vi "merFISH_create_tasks_list_TDMS.vi"(2 "Injection procedure empty?":bool, 3 "merFISH mode":u16, 4 "error in":errorcluster, 5 "merFISH path":path=path "E:/", 6 "Probe List Refnum":refnum<vi>, 7 "XY positions":dbl[][](array[numeric])) -> (0 "error out":errorcluster, 1 "refnum log file":refnum<file>)   [LabVIEW 2015]
uses:
  CONTROLS/Q_main_element.ctl
  GLOBAL/Global_MAIN.vi
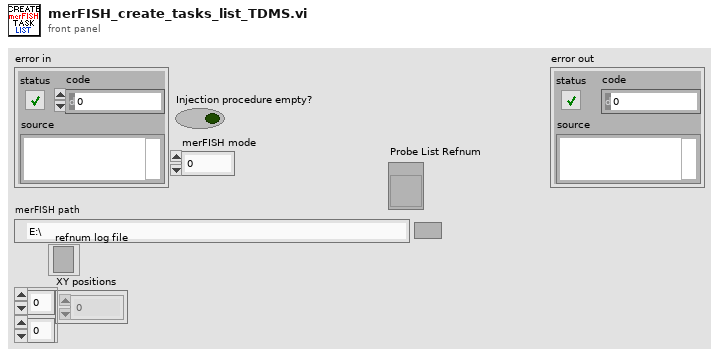
[diagram p1: front panel]
types:
  T1 = typedef "Q_main_element.ctl" = cluster{"variant":variant, "Instruction":enum16{"Main_idle", "Main_initialize", "Main_initialize_TDMS", "Main_initialize_Queue", "Main_error", "Main_DAQ_initialization_results", "Main_ASI_initialization_results", "Main_Piezo_initialization_results", "Main_Valve_initialization_results", "Main_Pump_initialization_results", "Main_CAMERA_initialization_results", "Main_FPGA_initialization_results", "Main_DAQ_error", "Main_ASI_error", "Main_Piezo_error", "Main_CAMERA_error", "Main_Valve_error", "Main_Pump_error", "Main_FPGA_error", "Main_start_acquiring", "Main_not_acquiring", "Main_acquiring", "Main_stop_acquiring", "Main_change_exposure", "Main_change_z_scan_parameters", "Main_define_ROI", "Main_define_mosaic", "Main_read_kinetic_time", "Main_cooler", "Main_read_temperature", "Main_save_XY", "Main_load_XY", "Main_discard_XY", "Main_move_to_XY", "Main_measure_QPD", "Main_autofocus_calibration", "Main_autofocus_initialization", "Main_autofocus_stop", "Main_save_PID", "Main_change_H_valve_position", "Main_two_way_valve", "Main_save_movie", "Main_init_single_scan", "Main_single_scan", "Main_stop_single_scan", "Main_merFISH_illumination_parameters", "Main_merFISH_buffer_probe_list", "Main_merFISH_injections_procedure", "Main_merFISH_save_setpoint", "Main_merFISH_DAPI_parameters", "Main_merFISH_Brightfield_parameters", "Main_merFISH_save_embryo_ROI", "Main_merFISH_init", "Main_merFISH_resume", "Main_merFISH_start_autofocus", "Main_merFISH_open_close_valve_merFISH", "Main_merFISH_open_close_valve_photobleaching", "Main_merFISH_hybridization", "Main_merFISH_move_to_ROI", "Main_merFISH_wait_stabilization", "Main_merFISH_move_to_REF", "Main_merFISH_scan", "Main_merFISH_photobleaching_injection", "Main_merFISH_photobleaching", "Main_merFISH_send_email", "Main_merFISH_close", "Main_STOP"}}
  T2 = enum16{"open", "replace", "create", "open or create", "replace or create", "replace or create with confirmation"}
  T3 = enum16{"Single ROIs & no injection", "Single ROIs & injections", "Embryos & no injection", "Embryos & injections"}
  T4 = cluster{"ROI #":i32, "Probe #":i32, "Folder# ":i32, "Embryo #":i32}
  T5 = enum16{"open", "open or create", "create or replace", "create", "open (read-only)"}
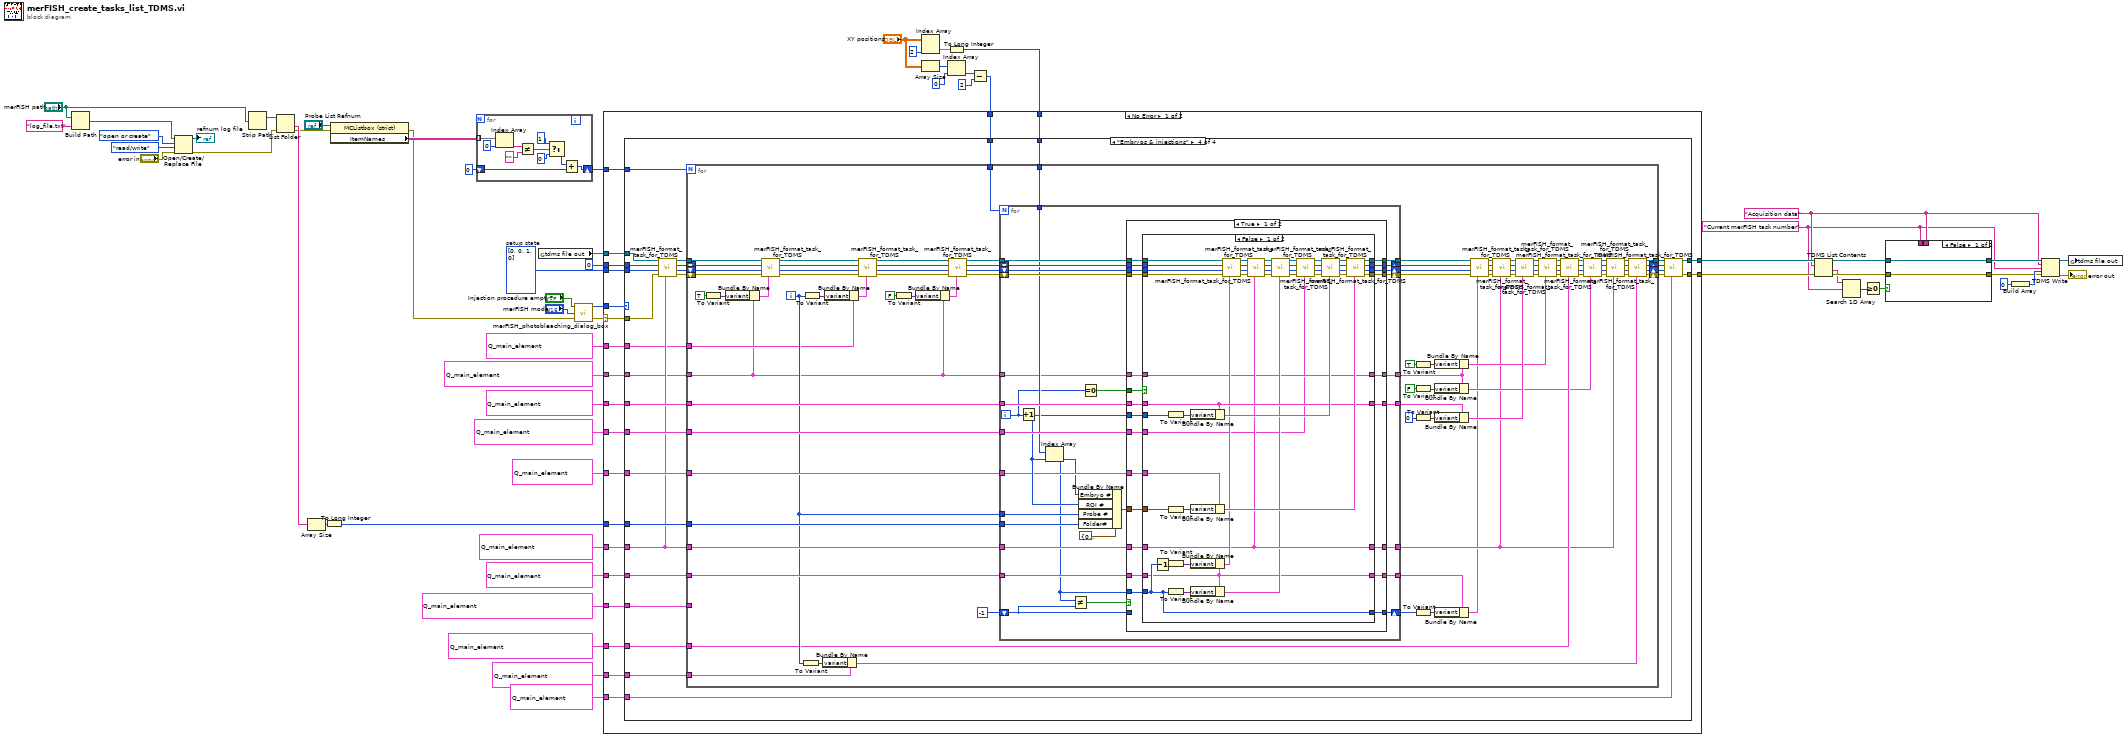
[diagram p0: block diagram]
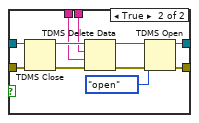
[diagram p2: hidden frame]
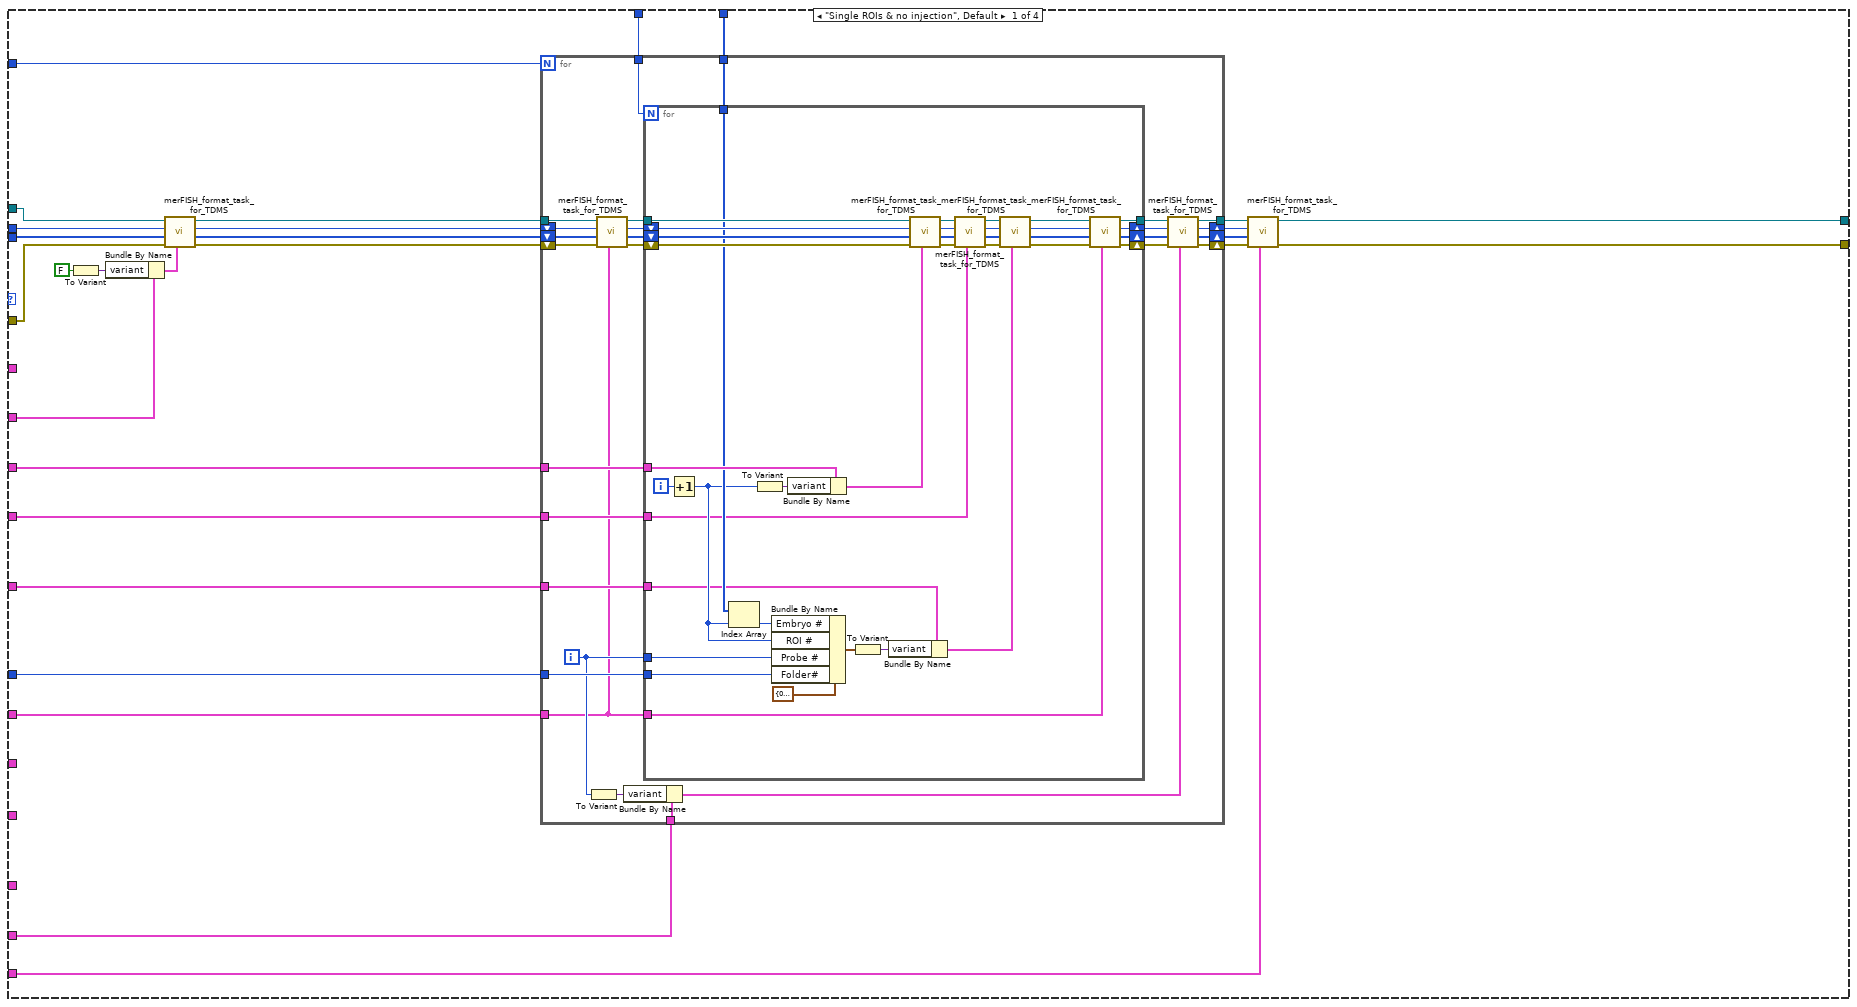
[diagram p3: hidden frame]
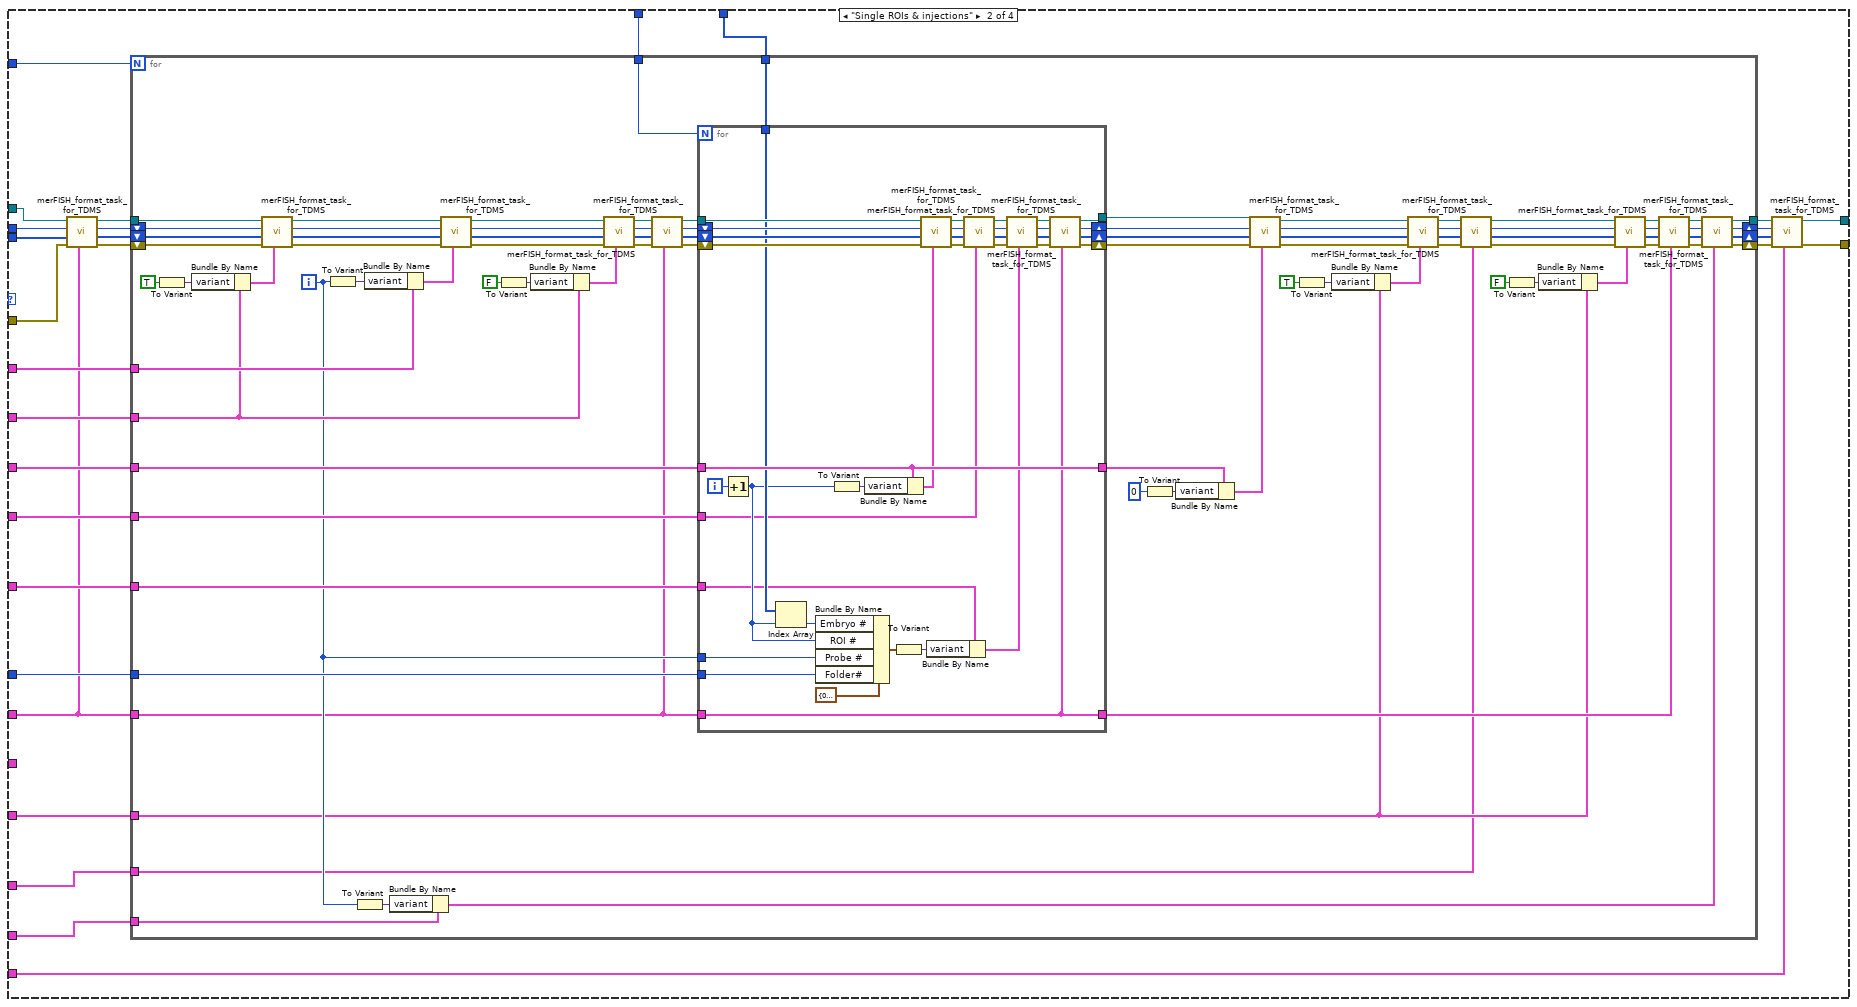
[diagram p4: hidden frame]
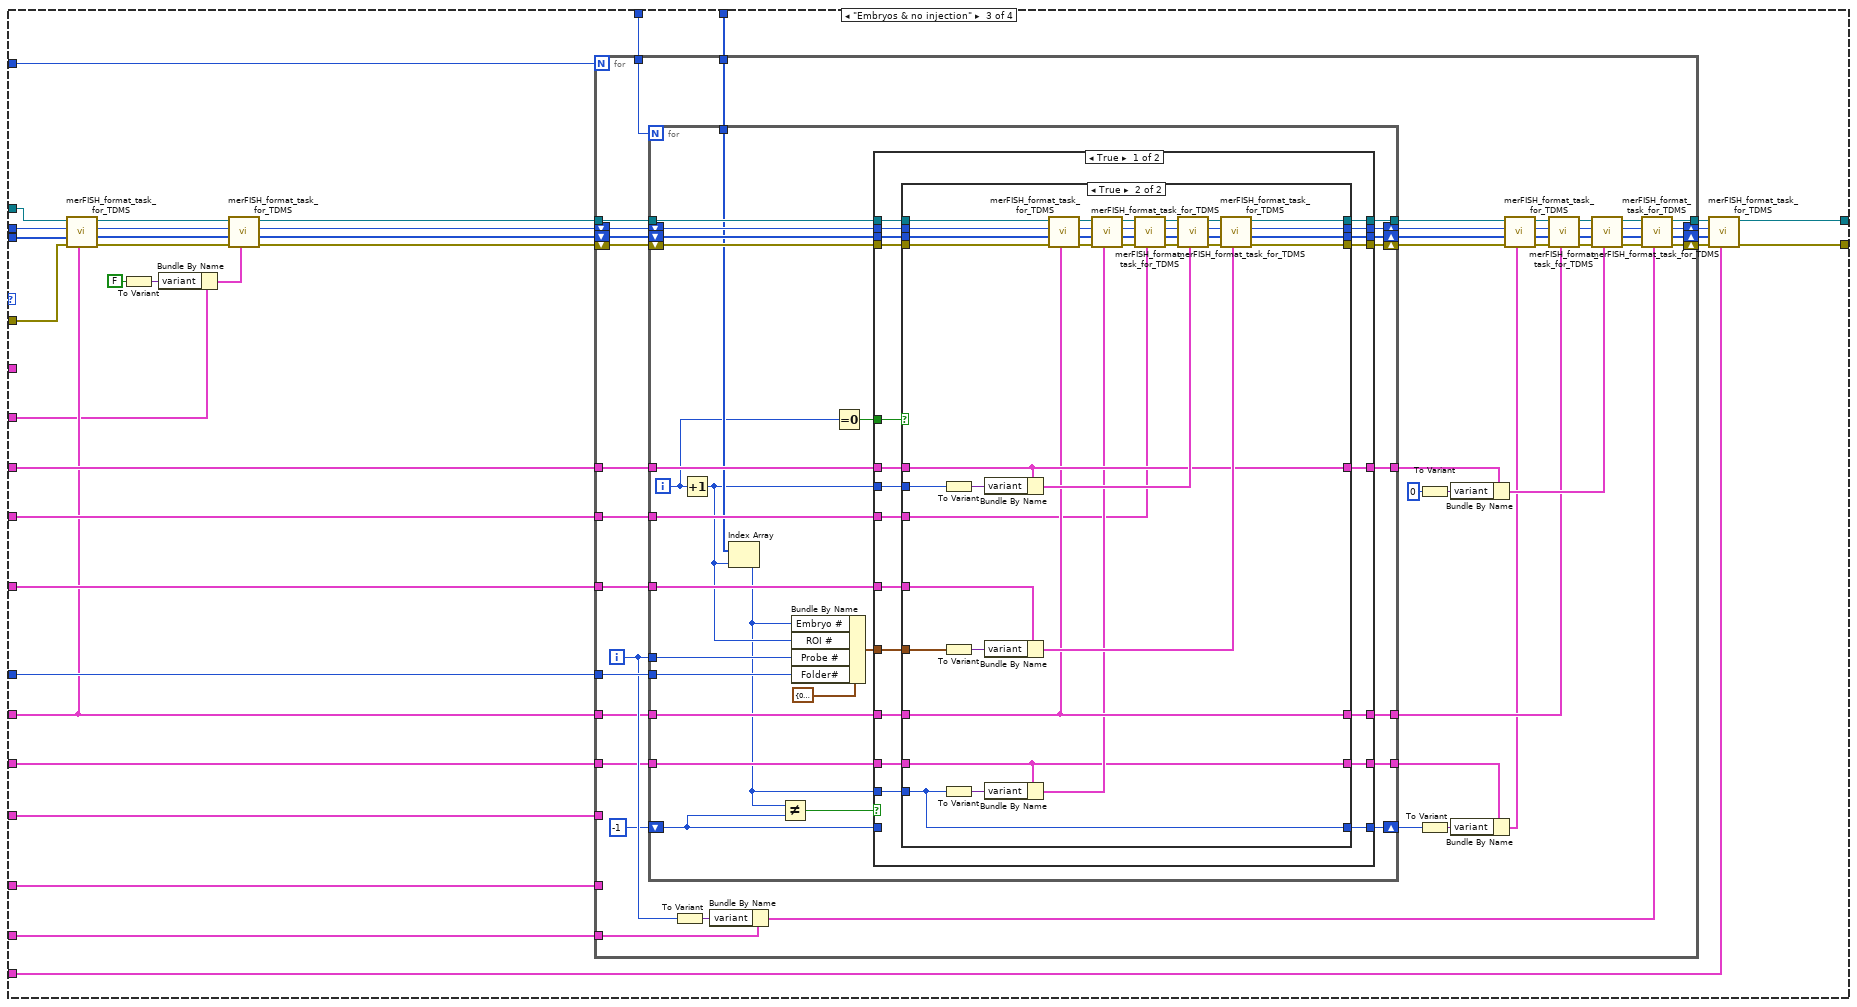
[diagram p5: hidden frame]
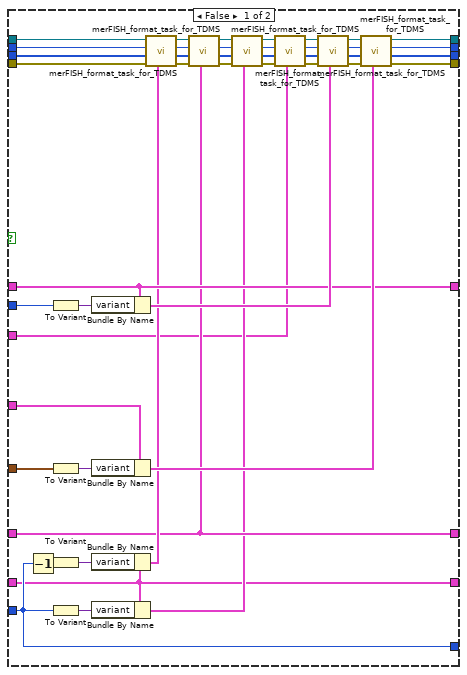
[diagram p6: hidden frame]
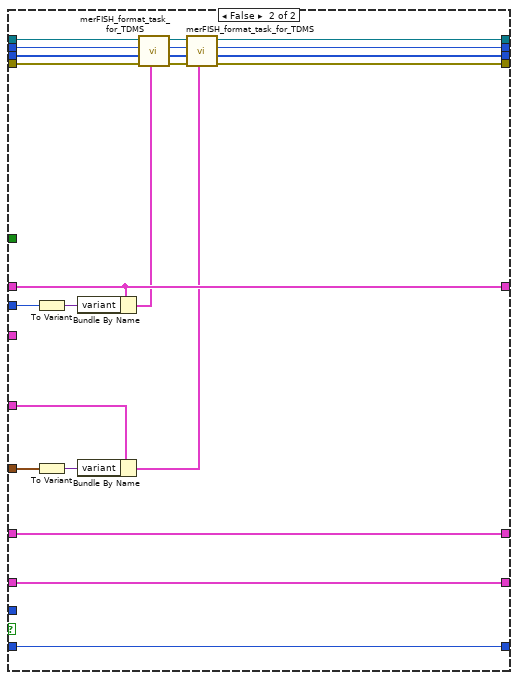
[diagram p7: hidden frame]
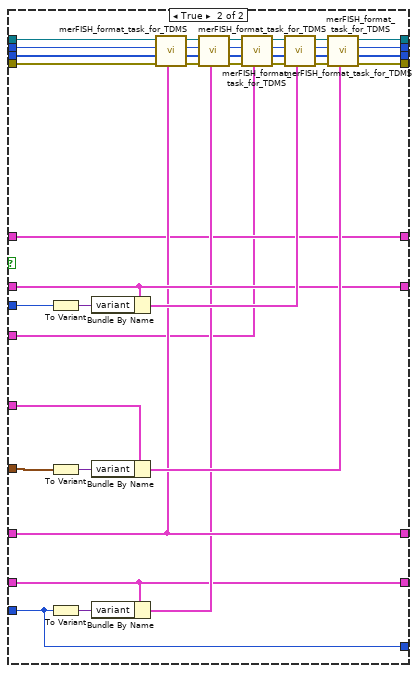
[diagram p8: hidden frame]
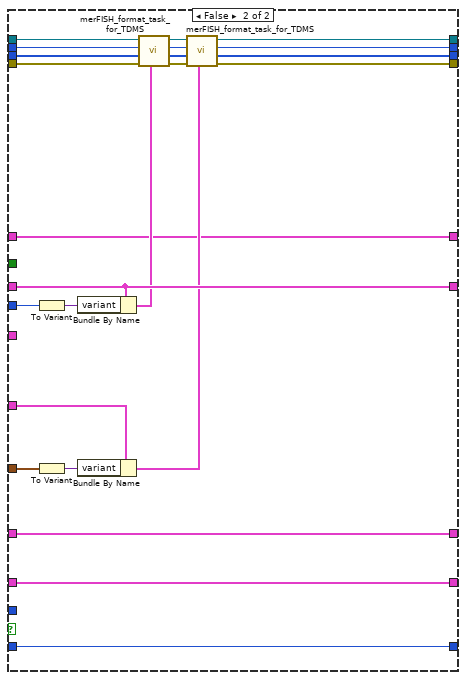
[diagram p9: hidden frame]
diagram:
  w13 = i32[] [0, 0, 1, 0]  # setup state
  w18 = "Current merFISH task number" ("group name in")
  w19 = "Acquisition data" ("group name in")
  n1 = Build Path(base path="merFISH path", name or relative path="log_file.txt") -> (appended path=w42:path)
  n2 = Open/Create/Replace File(file path (use dialog)=w42, error in="error in", operation (0:open)=T2."open or create", access (0:read/write)=enum16{"read/write", "read-only", "write-only"}."read/write") -> (refnum out=→"refnum log file":refnum<file>, error out=w37:errorcluster)  [unwired: 2 in, 1 out]
  n3 = Strip Path(path="merFISH path") -> (stripped path=w36:path)  [unwired: 1 out]
  n4 = List Folder(path=w36, error in=w37) -> (folder names=w50:string[], error out=w48:errorcluster)  [unwired: 2 in, 2 out]
  n5 = Array Size(array=w50) -> (size(s)=w49:i32)
  n6 = To Long Integer(number=w49) -> (32bit integer=w47:i32)
  n7 = property class="MCListbox (strict)"(reference="Probe List Refnum", error in=w48) -> (error out=w31:errorcluster, "ItemNames"=w53:string[][])  [unwired: 1 out]
  n8 = for {
    tunnel: w53 -> [w70] mode=indexing
    shift-right: [w63] -> w51
    shift-left: 0 ("f") -> [w61]
    n9 = Index Array(array=w70, index=0) -> (element=w68:string)
    n10 = Not Equal?(x=w68, y="") -> (x != y?=w66:bool)
    n11 = Select(t=1, s=w66, f=0) -> (s? t:f=w62:i32)
    n12 = Add(x=w62, y=w61) -> (x+y=w63:i32)
  }
  n13 = global read "Global_MAIN.vi" "tdms file out"() -> (w29:refnum<k34>)
  n14 = call "merFISH_photobleaching_dialog_box.vi"("error in"=w31, "merFISH mode"="merFISH mode", "Injection procedure empty?"="Injection procedure empty?") -> ("error out"=w35:errorcluster, "Which experiment?"=w34:T3)  [unwired: 1 in]
  n15 = Index Array(array="XY positions", index (col)=2 ("disabled index (col)")) -> (element=w4:dbl[])  [unwired: 1 in]
  n16 = Array Size(array="XY positions") -> (size(s)=w10:i32[])
  n17 = To Long Integer(number=w4) -> (32bit integer=w3:i32[])
  n18 = Index Array(array=w10, index=0) -> (element=w9:i32)
  n19 = Subtract(x=w9, y=2) -> (x-y=w7:i32)
  n20 = case shown="No Error" w35 {
    selector: w35 -> [w79 w850]
    tunnel: T1 {"variant"=variant, "Instruction"=enum."Main_merFISH_move_to_ROI"} ("element") -> [w92 _]
    tunnel: T1 {"variant"=variant, "Instruction"=enum."Main_merFISH_wait_stabilization"} ("element") -> [w91 _]
    tunnel: T1 {"variant"=variant, "Instruction"=enum."Main_merFISH_scan"} ("element") -> [w90 _]
    tunnel: T1 {"variant"=variant, "Instruction"=enum."Main_merFISH_close"} ("element") -> [w89 _]
    tunnel: T1 {"variant"=variant, "Instruction"=enum."Main_merFISH_start_autofocus"} ("element") -> [w88 _]
    tunnel: T1 {"variant"=variant, "Instruction"=enum."Main_merFISH_hybridization"} ("element") -> [w87 _]
    tunnel: w51 -> [w86 _]
    tunnel: w47 -> [w85 _]
    tunnel: T1 {"variant"=variant, "Instruction"=enum."Main_merFISH_open_close_valve_merFISH"} ("element") -> [w84 _]
    tunnel: w34 -> [w83 _]
    tunnel: T1 {"variant"=variant, "Instruction"=enum."Main_merFISH_photobleaching_injection"} ("element") -> [w82 _]
    tunnel: T1 {"variant"=variant, "Instruction"=enum."Main_merFISH_send_email"} ("element") -> [w81 _]
    tunnel: T1 {"variant"=variant, "Instruction"=enum."Main_merFISH_open_close_valve_photobleaching"} ("element") -> [w80 _]
    tunnel: 0 ("index") -> [w78 _]
    tunnel: [w77 w850] -> w21
    tunnel: w29 -> [w76 w849]
    tunnel: [w75 w849] -> w20
    tunnel: w13 -> [w74 _]
    tunnel: w7 -> [w73 _]
    tunnel: w3 -> [w72 _]
    tunnel: T1 {"variant"=variant, "Instruction"=enum."Main_merFISH_move_to_REF"} ("element") -> [w71 _]
    frame No Error {
      n21 = case shown="\"Embryos & injections\"" w83 {
        tunnel: w92 -> [w120 w208 w363 w593]
        tunnel: w91 -> [w119 w207 w362 w592]
        tunnel: w90 -> [w118 w206 w361 w591]
        tunnel: w89 -> [w111 w196 w353 w583]
        tunnel: w88 -> [w114 w201 w356 w586]
        tunnel: w87 -> [_ w210 _ w566]
        tunnel: w86 -> [w117 w211 w364 w594]
        tunnel: w85 -> [w116 w205 w360 w590]
        tunnel: w84 -> [w93 w209 w335 w567]
        tunnel: w82 -> [_ w203 w358 w588]
        tunnel: w81 -> [w115 w204 w359 w589]
        tunnel: w80 -> [_ w184 w343 w573]
        tunnel: w79 -> [w94 w202 w357 w587]
        tunnel: [w110 w195 w352 w582] -> w77
        tunnel: w78 -> [w99 w194 w351 w581]
        tunnel: w76 -> [w101 w193 w350 w580]
        tunnel: [w108 w190 w348 w578] -> w75
        tunnel: w74 -> [w95 w189 w347 w577]
        tunnel: w73 -> [w106 w186 w345 w575]
        tunnel: w72 -> [w105 w185 w344 w574]
        tunnel: w71 -> [_ _ w330 w572]
        frame "Single ROIs & no injection", Default {
          n22 = To Variant(anything=FALSE) -> (Variant=w104:variant)
          n23 = Bundle By Name(cluster=w93, "variant"=w104) -> (w102:T1)
          n24 = call "merFISH_format_task_for_TDMS.vi"("Task"=w102, "error in"=w94, "setup state"=w95, "Task number"=w99, "tdms file"=w101) -> ("error out"=w96:errorcluster, "setup state out"=w97:i32[], "Next task number"=w98:i32, "tdms file out"=w100:refnum<k34>)
          n25 = for {
            N: w117 -> [_]
            tunnel: w120 -> [w147]
            tunnel: w119 -> [w146]
            tunnel: w118 -> [w145]
            tunnel: w114 -> [w140]
            tunnel: w116 -> [w144]
            tunnel: w115 -> [w141]
            shift-right: [w134] -> w113
            shift-left: w98 -> [w124]
            shift-right: [w133] -> w112
            shift-left: w96 -> [w121]
            tunnel: w100 -> [w123]
            tunnel: [w130] -> w109
            shift-right: [w127] -> w107
            shift-left: w97 -> [w122]
            tunnel: w106 -> [w126]
            tunnel: w105 -> [w125]
            i -> [w142]
            n26 = To Variant(anything=w142) -> (Variant=w143:variant)
            n27 = call "merFISH_format_task_for_TDMS.vi"("Task"=w140, "error in"=w121, "setup state"=w122, "Task number"=w124, "tdms file"=w123) -> ("error out"=w138:errorcluster, "setup state out"=w129:i32[], "Next task number"=w139:i32, "tdms file out"=w132:refnum<k34>)
            n28 = Bundle By Name(cluster=w141, "variant"=w143) -> (w135:T1)
            n29 = for {
              N: w126 -> [_]
              tunnel: w147 -> [w182]
              tunnel: w146 -> [w148]
              tunnel: w145 -> [w157]
              tunnel: w140 -> [w171]
              tunnel: w142 -> [w180]
              tunnel: w144 -> [w179]
              shift-right: [w151] -> w137
              shift-left: w139 -> [w178]
              shift-right: [w149] -> w136
              shift-left: w138 -> [w177]
              tunnel: w132 -> [w170]
              tunnel: [w152] -> w131
              shift-right: [w150] -> w128
              shift-left: w129 -> [w167]
              tunnel: w125 -> [w163]
              i -> [w181]
              n30 = Increment(x=w181) -> (x+1=w162:i32)
              n31 = Index Array(array=w163, index=w162) -> (element=w161:i32)
              n32 = To Variant(anything=w162) -> (Variant=w183:variant)
              n33 = Bundle By Name(cluster=T4 {"ROI #"=0, "Probe #"=0, "Folder# "=0, "Embryo #"=0}, "Embryo #"=w161, "ROI #"=w162, "Probe #"=w180, "Folder#"=w179) -> (w160:T4)
              n34 = Bundle By Name(cluster=w182, "variant"=w183) -> (w176:T1)
              n35 = To Variant(anything=w160) -> (Variant=w158:variant)
              n36 = Bundle By Name(cluster=w157, "variant"=w158) -> (w159:T1)
              n37 = call "merFISH_format_task_for_TDMS.vi"("Task"=w176, "error in"=w177, "setup state"=w167, "Task number"=w178, "tdms file"=w170) -> ("error out"=w174:errorcluster, "setup state out"=w166:i32[], "Next task number"=w175:i32, "tdms file out"=w169:refnum<k34>)
              n38 = call "merFISH_format_task_for_TDMS.vi"("Task"=w148, "error in"=w174, "setup state"=w166, "Task number"=w175, "tdms file"=w169) -> ("error out"=w172:errorcluster, "setup state out"=w165:i32[], "Next task number"=w173:i32, "tdms file out"=w168:refnum<k34>)
              n39 = call "merFISH_format_task_for_TDMS.vi"("Task"=w159, "error in"=w172, "setup state"=w165, "Task number"=w173, "tdms file"=w168) -> ("error out"=w153:errorcluster, "setup state out"=w154:i32[], "Next task number"=w155:i32, "tdms file out"=w156:refnum<k34>)
              n40 = call "merFISH_format_task_for_TDMS.vi"("Task"=w171, "error in"=w153, "setup state"=w154, "Task number"=w155, "tdms file"=w156) -> ("error out"=w149:errorcluster, "setup state out"=w150:i32[], "Next task number"=w151:i32, "tdms file out"=w152:refnum<k34>)
            }
            n41 = call "merFISH_format_task_for_TDMS.vi"("Task"=w135, "error in"=w136, "setup state"=w128, "Task number"=w137, "tdms file"=w131) -> ("error out"=w133:errorcluster, "setup state out"=w127:i32[], "Next task number"=w134:i32, "tdms file out"=w130:refnum<k34>)
          }
          n42 = call "merFISH_format_task_for_TDMS.vi"("Task"=w111, "error in"=w112, "setup state"=w107, "Task number"=w113, "tdms file"=w109) -> ("error out"=w110:errorcluster, "tdms file out"=w108:refnum<k34>)  [unwired: 2 out]
        }
        frame "Single ROIs & injections" {
          n43 = call "merFISH_format_task_for_TDMS.vi"("Task"=w201, "error in"=w202, "setup state"=w189, "Task number"=w194, "tdms file"=w193) -> ("error out"=w199:errorcluster, "setup state out"=w188:i32[], "Next task number"=w200:i32, "tdms file out"=w192:refnum<k34>)
          n44 = for {
            N: w211 -> [_]
            tunnel: w208 -> [w293]
            tunnel: w207 -> [w292]
            tunnel: w206 -> [w291]
            tunnel: w201 -> [w261]
            tunnel: w210 -> [w284]
            tunnel: w205 -> [w289]
            tunnel: w209 -> [w279]
            tunnel: w184 -> [w213]
            tunnel: w204 -> [w274]
            tunnel: w203 -> [w212]
            shift-right: [w243] -> w197
            shift-left: w199 -> [w271]
            shift-right: [w242] -> w198
            shift-left: w200 -> [w272]
            tunnel: w192 -> [w241]
            tunnel: [w230] -> w191
            shift-right: [w218] -> w187
            shift-left: w188 -> [w229]
            tunnel: w186 -> [w217]
            tunnel: w185 -> [w216]
            i -> [w273]
            n45 = To Variant(anything=TRUE) -> (Variant=w288:variant)
            n46 = Bundle By Name(cluster=w279, "variant"=w288) -> (w270:T1)
            n47 = call "merFISH_format_task_for_TDMS.vi"("Task"=w270, "error in"=w271, "setup state"=w229, "Task number"=w272, "tdms file"=w241) -> ("error out"=w268:errorcluster, "setup state out"=w228:i32[], "Next task number"=w269:i32, "tdms file out"=w240:refnum<k34>)
            n48 = To Variant(anything=w273) -> (Variant=w290:variant)
            n49 = To Variant(anything=w273) -> (Variant=w275:variant)
            n50 = Bundle By Name(cluster=w284, "variant"=w290) -> (w267:T1)
            n51 = Bundle By Name(cluster=w274, "variant"=w275) -> (w215:T1)
            n52 = call "merFISH_format_task_for_TDMS.vi"("Task"=w267, "error in"=w268, "setup state"=w228, "Task number"=w269, "tdms file"=w240) -> ("error out"=w265:errorcluster, "setup state out"=w227:i32[], "Next task number"=w266:i32, "tdms file out"=w239:refnum<k34>)
            n53 = To Variant(anything=FALSE) -> (Variant=w285:variant)
            n54 = Bundle By Name(cluster=w279, "variant"=w285) -> (w264:T1)
            n55 = call "merFISH_format_task_for_TDMS.vi"("Task"=w264, "error in"=w265, "setup state"=w227, "Task number"=w266, "tdms file"=w239) -> ("error out"=w262:errorcluster, "setup state out"=w226:i32[], "Next task number"=w263:i32, "tdms file out"=w238:refnum<k34>)
            n56 = call "merFISH_format_task_for_TDMS.vi"("Task"=w261, "error in"=w262, "setup state"=w226, "Task number"=w263, "tdms file"=w238) -> ("error out"=w260:errorcluster, "setup state out"=w225:i32[], "Next task number"=w259:i32, "tdms file out"=w237:refnum<k34>)
            n57 = for {
              N: w217 -> [_]
              tunnel: w293 -> [w325]
              tunnel: w292 -> [w294]
              tunnel: w291 -> [w301]
              tunnel: w261 -> [w317]
              tunnel: w273 -> [w327]
              tunnel: w289 -> [w326]
              tunnel: [w325] -> w277
              tunnel: [w317] -> w248
              shift-right: [w315] -> w258
              shift-left: w259 -> [w324]
              shift-right: [w316] -> w257
              shift-left: w260 -> [w323]
              tunnel: w237 -> [w314]
              tunnel: [w311] -> w236
              shift-right: [w307] -> w224
              shift-left: w225 -> [w310]
              tunnel: w216 -> [w304]
              i -> [w328]
              n58 = Increment(x=w328) -> (x+1=w303:i32)
              n59 = Index Array(array=w304, index=w303) -> (element=w305:i32)
              n60 = Bundle By Name(cluster=T4 {"ROI #"=0, "Probe #"=0, "Folder# "=0, "Embryo #"=0}, "Embryo #"=w305, "ROI #"=w303, "Probe #"=w327, "Folder#"=w326) -> (w300:T4)
              n61 = To Variant(anything=w303) -> (Variant=w329:variant)
              n62 = Bundle By Name(cluster=w325, "variant"=w329) -> (w322:T1)
              n63 = To Variant(anything=w300) -> (Variant=w302:variant)
              n64 = call "merFISH_format_task_for_TDMS.vi"("Task"=w322, "error in"=w323, "setup state"=w310, "Task number"=w324, "tdms file"=w314) -> ("error out"=w320:errorcluster, "setup state out"=w309:i32[], "Next task number"=w321:i32, "tdms file out"=w313:refnum<k34>)
              n65 = Bundle By Name(cluster=w301, "variant"=w302) -> (w299:T1)
              n66 = call "merFISH_format_task_for_TDMS.vi"("Task"=w294, "error in"=w320, "setup state"=w309, "Task number"=w321, "tdms file"=w313) -> ("error out"=w319:errorcluster, "setup state out"=w308:i32[], "Next task number"=w318:i32, "tdms file out"=w312:refnum<k34>)
              n67 = call "merFISH_format_task_for_TDMS.vi"("Task"=w299, "error in"=w319, "setup state"=w308, "Task number"=w318, "tdms file"=w312) -> ("error out"=w295:errorcluster, "setup state out"=w296:i32[], "Next task number"=w297:i32, "tdms file out"=w298:refnum<k34>)
              n68 = call "merFISH_format_task_for_TDMS.vi"("Task"=w317, "error in"=w295, "setup state"=w296, "Task number"=w297, "tdms file"=w298) -> ("error out"=w316:errorcluster, "setup state out"=w307:i32[], "Next task number"=w315:i32, "tdms file out"=w311:refnum<k34>)
            }
            n69 = To Variant(anything=0) -> (Variant=w278:variant)
            n70 = Bundle By Name(cluster=w277, "variant"=w278) -> (w256:T1)
            n71 = call "merFISH_format_task_for_TDMS.vi"("Task"=w256, "error in"=w257, "setup state"=w224, "Task number"=w258, "tdms file"=w236) -> ("error out"=w254:errorcluster, "setup state out"=w223:i32[], "Next task number"=w255:i32, "tdms file out"=w235:refnum<k34>)
            n72 = To Variant(anything=TRUE) -> (Variant=w283:variant)
            n73 = Bundle By Name(cluster=w213, "variant"=w283) -> (w214:T1)
            n74 = call "merFISH_format_task_for_TDMS.vi"("Task"=w214, "error in"=w254, "setup state"=w223, "Task number"=w255, "tdms file"=w235) -> ("error out"=w253:errorcluster, "setup state out"=w222:i32[], "Next task number"=w252:i32, "tdms file out"=w234:refnum<k34>)
            n75 = call "merFISH_format_task_for_TDMS.vi"("Task"=w212, "error in"=w253, "setup state"=w222, "Task number"=w252, "tdms file"=w234) -> ("error out"=w250:errorcluster, "setup state out"=w221:i32[], "Next task number"=w251:i32, "tdms file out"=w233:refnum<k34>)
            n76 = To Variant(anything=FALSE) -> (Variant=w280:variant)
            n77 = Bundle By Name(cluster=w213, "variant"=w280) -> (w249:T1)
            n78 = call "merFISH_format_task_for_TDMS.vi"("Task"=w249, "error in"=w250, "setup state"=w221, "Task number"=w251, "tdms file"=w233) -> ("error out"=w247:errorcluster, "setup state out"=w220:i32[], "Next task number"=w246:i32, "tdms file out"=w232:refnum<k34>)
            n79 = call "merFISH_format_task_for_TDMS.vi"("Task"=w248, "error in"=w247, "setup state"=w220, "Task number"=w246, "tdms file"=w232) -> ("error out"=w244:errorcluster, "setup state out"=w219:i32[], "Next task number"=w245:i32, "tdms file out"=w231:refnum<k34>)
            n80 = call "merFISH_format_task_for_TDMS.vi"("Task"=w215, "error in"=w244, "setup state"=w219, "Task number"=w245, "tdms file"=w231) -> ("error out"=w243:errorcluster, "setup state out"=w218:i32[], "Next task number"=w242:i32, "tdms file out"=w230:refnum<k34>)
          }
          n81 = call "merFISH_format_task_for_TDMS.vi"("Task"=w196, "error in"=w197, "setup state"=w187, "Task number"=w198, "tdms file"=w191) -> ("error out"=w195:errorcluster, "tdms file out"=w190:refnum<k34>)  [unwired: 2 out]
        }
        frame "Embryos & no injection" {
          n82 = call "merFISH_format_task_for_TDMS.vi"("Task"=w356, "error in"=w357, "setup state"=w347, "Task number"=w351, "tdms file"=w350) -> ("error out"=w336:errorcluster, "setup state out"=w337:i32[], "Next task number"=w338:i32, "tdms file out"=w339:refnum<k34>)
          n83 = To Variant(anything=FALSE) -> (Variant=w342:variant)
          n84 = Bundle By Name(cluster=w335, "variant"=w342) -> (w340:T1)
          n85 = call "merFISH_format_task_for_TDMS.vi"("Task"=w340, "error in"=w336, "setup state"=w337, "Task number"=w338, "tdms file"=w339) -> ("error out"=w331:errorcluster, "setup state out"=w332:i32[], "Next task number"=w333:i32, "tdms file out"=w334:refnum<k34>)
          n86 = for {
            N: w364 -> [_]
            tunnel: w363 -> [w410]
            tunnel: w362 -> [w409]
            tunnel: w361 -> [w408]
            tunnel: w356 -> [w400]
            tunnel: w360 -> [w407]
            tunnel: w343 -> [_]
            tunnel: w359 -> [w402]
            tunnel: w358 -> [_]
            shift-right: [w397] -> w354
            shift-left: w331 -> [w387]
            shift-right: [w396] -> w355
            shift-left: w333 -> [w389]
            tunnel: [w395] -> w349
            shift-right: [w394] -> w346
            shift-left: w332 -> [w388]
            tunnel: w345 -> [w393]
            tunnel: w344 -> [w392]
            tunnel: w334 -> [w390]
            tunnel: w330 -> [w377]
            i -> [w401]
            n87 = for {
              N: w393 -> [_]
              tunnel: w410 -> [w435]
              tunnel: w409 -> [w436]
              tunnel: w408 -> [w423]
              tunnel: w400 -> [w432]
              tunnel: w401 -> [w438]
              tunnel: w407 -> [w437]
              tunnel: [w418] -> w405
              tunnel: [w417] -> w398
              shift-right: [w430] -> w371
              shift-left: w389 -> [w434]
              shift-right: [w431] -> w369
              shift-left: w387 -> [w433]
              tunnel: w390 -> [w429]
              tunnel: [w428] -> w372
              shift-right: [w426] -> w370
              shift-left: w388 -> [w427]
              tunnel: w392 -> [w424]
              shift-right: [w415] -> w367
              shift-left: -1 ("element") -> [w420]
              tunnel: w377 -> [w416]
              tunnel: [w411] -> w365
              i -> [w414]
              n88 = Increment(x=w414) -> (x+1=w413:i32)
              n89 = Index Array(array=w424, index=w413) -> (element=w412:i32)
              n90 = Not Equal?(x=w412, y=w420) -> (x != y?=w419:bool)
              n91 = Bundle By Name(cluster=T4 {"ROI #"=0, "Probe #"=0, "Folder# "=0, "Embryo #"=0}, "Embryo #"=w412, "ROI #"=w413, "Probe #"=w438, "Folder#"=w437) -> (w422:T4)
              n92 = Equal To 0?(x=w414) -> (x = 0?=w421:bool)
              n93 = case shown="True" w419 {
                tunnel: w436 -> [w459 _]
                tunnel: w435 -> [w447 w558]
                tunnel: w434 -> [w458 w565]
                tunnel: w433 -> [w457 w564]
                tunnel: w432 -> [w446 w557]
                tunnel: [w456 w549] -> w431
                tunnel: [w455 w551] -> w430
                tunnel: w429 -> [w454 w563]
                tunnel: [w453 w552] -> w428
                tunnel: w427 -> [w452 w562]
                tunnel: [w451 w550] -> w426
                tunnel: w413 -> [w450 w561]
                tunnel: w423 -> [w449 w560]
                tunnel: w422 -> [w448 w559]
                tunnel: w421 -> [w445 _]
                tunnel: w420 -> [_ w544]
                tunnel: [w444 w558] -> w418
                tunnel: [w443 w557] -> w417
                tunnel: w416 -> [w441 w543]
                tunnel: w412 -> [w442 _]
                tunnel: [w440 w544] -> w415
                tunnel: [w439 w543] -> w411
                frame True {
                  n94 = case shown="True" w445 {
                    tunnel: w459 -> [w461 w506]
                    tunnel: w458 -> [w495 w533]
                    tunnel: w457 -> [w493 w531]
                    tunnel: [w462 w507] -> w456
                    tunnel: [w464 w509] -> w455
                    tunnel: w454 -> [w496 w534]
                    tunnel: [w465 w510] -> w453
                    tunnel: w452 -> [w494 w532]
                    tunnel: [w463 w508] -> w451
                    tunnel: w450 -> [w502 w540]
                    tunnel: w449 -> [w500 w538]
                    tunnel: w448 -> [w499 w537]
                    tunnel: w447 -> [w497 w535]
                    tunnel: w446 -> [w484 w529]
                    tunnel: [w497 w535] -> w444
                    tunnel: [w484 w529] -> w443
                    tunnel: w442 -> [w478 w523]
                    tunnel: w441 -> [w460 w505]
                    tunnel: [w478 w523] -> w440
                    tunnel: [w460 w505] -> w439
                    frame False {
                      n95 = Decrement(x=w478) -> (x-1=w492:i32)
                      n96 = To Variant(anything=w502) -> (Variant=w504:variant)
                      n97 = To Variant(anything=w499) -> (Variant=w501:variant)
                      n98 = To Variant(anything=w492) -> (Variant=w491:variant)
                      n99 = To Variant(anything=w478) -> (Variant=w490:variant)
                      n100 = Bundle By Name(cluster=w497, "variant"=w504) -> (w503:T1)
                      n101 = Bundle By Name(cluster=w500, "variant"=w501) -> (w498:T1)
                      n102 = Bundle By Name(cluster=w460, "variant"=w491) -> (w489:T1)
                      n103 = Bundle By Name(cluster=w460, "variant"=w490) -> (w479:T1)
                      n104 = call "merFISH_format_task_for_TDMS.vi"("Task"=w489, "error in"=w493, "setup state"=w494, "Task number"=w495, "tdms file"=w496) -> ("error out"=w485:errorcluster, "setup state out"=w486:i32[], "Next task number"=w487:i32, "tdms file out"=w488:refnum<k34>)
                      n105 = call "merFISH_format_task_for_TDMS.vi"("Task"=w484, "error in"=w485, "setup state"=w486, "Task number"=w487, "tdms file"=w488) -> ("error out"=w483:errorcluster, "setup state out"=w482:i32[], "Next task number"=w481:i32, "tdms file out"=w480:refnum<k34>)
                      n106 = call "merFISH_format_task_for_TDMS.vi"("Task"=w479, "error in"=w483, "setup state"=w482, "Task number"=w481, "tdms file"=w480) -> ("error out"=w474:errorcluster, "setup state out"=w475:i32[], "Next task number"=w476:i32, "tdms file out"=w477:refnum<k34>)
                      n107 = call "merFISH_format_task_for_TDMS.vi"("Task"=w461, "error in"=w474, "setup state"=w475, "Task number"=w476, "tdms file"=w477) -> ("error out"=w470:errorcluster, "setup state out"=w471:i32[], "Next task number"=w472:i32, "tdms file out"=w473:refnum<k34>)
                      n108 = call "merFISH_format_task_for_TDMS.vi"("Task"=w503, "error in"=w470, "setup state"=w471, "Task number"=w472, "tdms file"=w473) -> ("error out"=w466:errorcluster, "setup state out"=w467:i32[], "Next task number"=w468:i32, "tdms file out"=w469:refnum<k34>)
                      n109 = call "merFISH_format_task_for_TDMS.vi"("Task"=w498, "error in"=w466, "setup state"=w467, "Task number"=w468, "tdms file"=w469) -> ("error out"=w462:errorcluster, "setup state out"=w463:i32[], "Next task number"=w464:i32, "tdms file out"=w465:refnum<k34>)
                    }
                    frame True {
                      n110 = To Variant(anything=w540) -> (Variant=w542:variant)
                      n111 = To Variant(anything=w537) -> (Variant=w539:variant)
                      n112 = To Variant(anything=w523) -> (Variant=w530:variant)
                      n113 = Bundle By Name(cluster=w535, "variant"=w542) -> (w541:T1)
                      n114 = Bundle By Name(cluster=w538, "variant"=w539) -> (w536:T1)
                      n115 = Bundle By Name(cluster=w505, "variant"=w530) -> (w524:T1)
                      n116 = call "merFISH_format_task_for_TDMS.vi"("Task"=w529, "error in"=w531, "setup state"=w532, "Task number"=w533, "tdms file"=w534) -> ("error out"=w528:errorcluster, "setup state out"=w527:i32[], "Next task number"=w526:i32, "tdms file out"=w525:refnum<k34>)
                      n117 = call "merFISH_format_task_for_TDMS.vi"("Task"=w524, "error in"=w528, "setup state"=w527, "Task number"=w526, "tdms file"=w525) -> ("error out"=w519:errorcluster, "setup state out"=w520:i32[], "Next task number"=w521:i32, "tdms file out"=w522:refnum<k34>)
                      n118 = call "merFISH_format_task_for_TDMS.vi"("Task"=w506, "error in"=w519, "setup state"=w520, "Task number"=w521, "tdms file"=w522) -> ("error out"=w518:errorcluster, "setup state out"=w517:i32[], "Next task number"=w516:i32, "tdms file out"=w515:refnum<k34>)
                      n119 = call "merFISH_format_task_for_TDMS.vi"("Task"=w541, "error in"=w518, "setup state"=w517, "Task number"=w516, "tdms file"=w515) -> ("error out"=w511:errorcluster, "setup state out"=w512:i32[], "Next task number"=w513:i32, "tdms file out"=w514:refnum<k34>)
                      n120 = call "merFISH_format_task_for_TDMS.vi"("Task"=w536, "error in"=w511, "setup state"=w512, "Task number"=w513, "tdms file"=w514) -> ("error out"=w507:errorcluster, "setup state out"=w508:i32[], "Next task number"=w509:i32, "tdms file out"=w510:refnum<k34>)
                    }
                  }
                }
                frame False {
                  n121 = To Variant(anything=w561) -> (Variant=w556:variant)
                  n122 = To Variant(anything=w559) -> (Variant=w554:variant)
                  n123 = Bundle By Name(cluster=w558, "variant"=w556) -> (w555:T1)
                  n124 = Bundle By Name(cluster=w560, "variant"=w554) -> (w553:T1)
                  n125 = call "merFISH_format_task_for_TDMS.vi"("Task"=w555, "error in"=w564, "setup state"=w562, "Task number"=w565, "tdms file"=w563) -> ("error out"=w545:errorcluster, "setup state out"=w546:i32[], "Next task number"=w547:i32, "tdms file out"=w548:refnum<k34>)
                  n126 = call "merFISH_format_task_for_TDMS.vi"("Task"=w553, "error in"=w545, "setup state"=w546, "Task number"=w547, "tdms file"=w548) -> ("error out"=w549:errorcluster, "setup state out"=w550:i32[], "Next task number"=w551:i32, "tdms file out"=w552:refnum<k34>)
                }
              }
            }
            n127 = To Variant(anything=w401) -> (Variant=w403:variant)
            n128 = Bundle By Name(cluster=w402, "variant"=w403) -> (w391:T1)
            n129 = To Variant(anything=0) -> (Variant=w406:variant)
            n130 = To Variant(anything=w367) -> (Variant=w368:variant)
            n131 = Bundle By Name(cluster=w405, "variant"=w406) -> (w399:T1)
            n132 = Bundle By Name(cluster=w365, "variant"=w368) -> (w366:T1)
            n133 = call "merFISH_format_task_for_TDMS.vi"("Task"=w366, "error in"=w369, "setup state"=w370, "Task number"=w371, "tdms file"=w372) -> ("error out"=w376:errorcluster, "setup state out"=w375:i32[], "Next task number"=w374:i32, "tdms file out"=w373:refnum<k34>)
            n134 = call "merFISH_format_task_for_TDMS.vi"("Task"=w398, "error in"=w376, "setup state"=w375, "Task number"=w374, "tdms file"=w373) -> ("error out"=w383:errorcluster, "setup state out"=w384:i32[], "Next task number"=w385:i32, "tdms file out"=w386:refnum<k34>)
            n135 = call "merFISH_format_task_for_TDMS.vi"("Task"=w399, "error in"=w383, "setup state"=w384, "Task number"=w385, "tdms file"=w386) -> ("error out"=w379:errorcluster, "setup state out"=w380:i32[], "Next task number"=w381:i32, "tdms file out"=w382:refnum<k34>)
            n136 = call "merFISH_format_task_for_TDMS.vi"("Task"=w391, "error in"=w379, "setup state"=w380, "Task number"=w381, "tdms file"=w382) -> ("error out"=w397:errorcluster, "setup state out"=w394:i32[], "Next task number"=w396:i32, "tdms file out"=w395:refnum<k34>)
          }
          n137 = call "merFISH_format_task_for_TDMS.vi"("Task"=w353, "error in"=w354, "setup state"=w346, "Task number"=w355, "tdms file"=w349) -> ("error out"=w352:errorcluster, "tdms file out"=w348:refnum<k34>)  [unwired: 2 out]
        }
        frame "Embryos & injections" {
          n138 = call "merFISH_format_task_for_TDMS.vi"("Task"=w586, "error in"=w587, "setup state"=w577, "Task number"=w581, "tdms file"=w580) -> ("error out"=w568:errorcluster, "setup state out"=w569:i32[], "Next task number"=w570:i32, "tdms file out"=w571:refnum<k34>)
          n139 = for {
            N: w594 -> [_]
            tunnel: w593 -> [w686]
            tunnel: w592 -> [w685]
            tunnel: w591 -> [w684]
            tunnel: w586 -> [w677]
            tunnel: w590 -> [w683]
            tunnel: w573 -> [_]
            tunnel: w589 -> [w678]
            tunnel: w588 -> [w625]
            shift-right: [w675] -> w584
            shift-left: w568 -> [w656]
            shift-right: [w674] -> w585
            shift-left: w570 -> [w658]
            tunnel: [w673] -> w579
            shift-right: [w672] -> w576
            shift-left: w569 -> [w657]
            tunnel: w575 -> [w671]
            tunnel: w574 -> [w670]
            tunnel: w571 -> [w659]
            tunnel: w572 -> [w663]
            tunnel: w567 -> [w630]
            tunnel: w566 -> [w648]
            i -> [w649]
            n140 = To Variant(anything=TRUE) -> (Variant=w662:variant)
            n141 = Bundle By Name(cluster=w630, "variant"=w662) -> (w660:T1)
            n142 = call "merFISH_format_task_for_TDMS.vi"("Task"=w660, "error in"=w656, "setup state"=w657, "Task number"=w658, "tdms file"=w659) -> ("error out"=w650:errorcluster, "setup state out"=w651:i32[], "Next task number"=w652:i32, "tdms file out"=w653:refnum<k34>)
            n143 = To Variant(anything=w649) -> (Variant=w679:variant)
            n144 = To Variant(anything=w649) -> (Variant=w654:variant)
            n145 = Bundle By Name(cluster=w678, "variant"=w679) -> (w669:T1)
            n146 = Bundle By Name(cluster=w648, "variant"=w654) -> (w655:T1)
            n147 = call "merFISH_format_task_for_TDMS.vi"("Task"=w655, "error in"=w650, "setup state"=w651, "Task number"=w652, "tdms file"=w653) -> ("error out"=w642:errorcluster, "setup state out"=w643:i32[], "Next task number"=w644:i32, "tdms file out"=w645:refnum<k34>)
            n148 = To Variant(anything=FALSE) -> (Variant=w646:variant)
            n149 = Bundle By Name(cluster=w630, "variant"=w646) -> (w641:T1)
            n150 = call "merFISH_format_task_for_TDMS.vi"("Task"=w641, "error in"=w642, "setup state"=w643, "Task number"=w644, "tdms file"=w645) -> ("error out"=w637:errorcluster, "setup state out"=w638:i32[], "Next task number"=w639:i32, "tdms file out"=w640:refnum<k34>)
            n151 = for {
              N: w671 -> [_]
              tunnel: w686 -> [w713]
              tunnel: w685 -> [w714]
              tunnel: w684 -> [w700]
              tunnel: w677 -> [w710]
              tunnel: w649 -> [w716]
              tunnel: w683 -> [w715]
              tunnel: [w695] -> w681
              tunnel: [w694] -> w611
              shift-right: [w708] -> w602
              shift-left: w639 -> [w712]
              shift-right: [w709] -> w600
              shift-left: w637 -> [w711]
              tunnel: w640 -> [w707]
              tunnel: [w706] -> w603
              shift-right: [w704] -> w601
              shift-left: w638 -> [w705]
              tunnel: w670 -> [w702]
              shift-right: [w690] -> w605
              shift-left: -1 ("element") -> [w697]
              tunnel: w663 -> [w693]
              tunnel: w630 -> [w692]
              tunnel: [w691] -> w621
              tunnel: [w689] -> w599
              i -> [w688]
              n152 = Increment(x=w688) -> (x+1=w701:i32)
              n153 = Index Array(array=w702, index=w701) -> (element=w687:i32)
              n154 = Not Equal?(x=w687, y=w697) -> (x != y?=w696:bool)
              n155 = Bundle By Name(cluster=T4 {"ROI #"=0, "Probe #"=0, "Folder# "=0, "Embryo #"=0}, "Embryo #"=w687, "ROI #"=w701, "Probe #"=w716, "Folder#"=w715) -> (w699:T4)
              n156 = Equal To 0?(x=w688) -> (x = 0?=w698:bool)
              n157 = case shown="True" w696 {
                tunnel: w714 -> [w739 _]
                tunnel: w713 -> [w727 w841]
                tunnel: w712 -> [w738 w848]
                tunnel: w711 -> [w737 w847]
                tunnel: w710 -> [w726 w840]
                tunnel: [w736 w832] -> w709
                tunnel: [w735 w834] -> w708
                tunnel: w707 -> [w734 w846]
                tunnel: [w733 w835] -> w706
                tunnel: w705 -> [w732 w845]
                tunnel: [w731 w833] -> w704
                tunnel: w701 -> [w730 w844]
                tunnel: w700 -> [w729 w843]
                tunnel: w699 -> [w728 w842]
                tunnel: w698 -> [w725 _]
                tunnel: w697 -> [_ w826]
                tunnel: [w724 w841] -> w695
                tunnel: [w723 w840] -> w694
                tunnel: w693 -> [w721 w825]
                tunnel: w687 -> [w722 _]
                tunnel: w692 -> [w720 w827]
                tunnel: [w719 w827] -> w691
                tunnel: [w718 w826] -> w690
                tunnel: [w717 w825] -> w689
                frame True {
                  n158 = case shown="False" w725 {
                    tunnel: w739 -> [w757 w803]
                    tunnel: w738 -> [w776 w815]
                    tunnel: w737 -> [w774 w813]
                    tunnel: [w753 w799] -> w736
                    tunnel: [w755 w801] -> w735
                    tunnel: w734 -> [w777 w816]
                    tunnel: [w756 w802] -> w733
                    tunnel: w732 -> [w775 w814]
                    tunnel: [w754 w800] -> w731
                    tunnel: w730 -> [w783 w822]
                    tunnel: w729 -> [w781 w820]
                    tunnel: w728 -> [w780 w819]
                    tunnel: w727 -> [w778 w817]
                    tunnel: w726 -> [w765 w811]
                    tunnel: [w778 w817] -> w724
                    tunnel: [w765 w811] -> w723
                    tunnel: w722 -> [w758 w804]
                    tunnel: w721 -> [w752 w798]
                    tunnel: w720 -> [w759 w805]
                    tunnel: [w759 w805] -> w719
                    tunnel: [w758 w804] -> w718
                    tunnel: [w752 w798] -> w717
                    frame False {
                      n159 = Decrement(x=w758) -> (x-1=w773:i32)
                      n160 = To Variant(anything=w783) -> (Variant=w785:variant)
                      n161 = To Variant(anything=w780) -> (Variant=w782:variant)
                      n162 = To Variant(anything=w773) -> (Variant=w772:variant)
                      n163 = To Variant(anything=w758) -> (Variant=w771:variant)
                      n164 = Bundle By Name(cluster=w778, "variant"=w785) -> (w784:T1)
                      n165 = Bundle By Name(cluster=w781, "variant"=w782) -> (w779:T1)
                      n166 = Bundle By Name(cluster=w752, "variant"=w772) -> (w770:T1)
                      n167 = Bundle By Name(cluster=w752, "variant"=w771) -> (w760:T1)
                      n168 = call "merFISH_format_task_for_TDMS.vi"("Task"=w770, "error in"=w774, "setup state"=w775, "Task number"=w776, "tdms file"=w777) -> ("error out"=w766:errorcluster, "setup state out"=w767:i32[], "Next task number"=w768:i32, "tdms file out"=w769:refnum<k34>)
                      n169 = call "merFISH_format_task_for_TDMS.vi"("Task"=w765, "error in"=w766, "setup state"=w767, "Task number"=w768, "tdms file"=w769) -> ("error out"=w764:errorcluster, "setup state out"=w763:i32[], "Next task number"=w762:i32, "tdms file out"=w761:refnum<k34>)
                      n170 = call "merFISH_format_task_for_TDMS.vi"("Task"=w760, "error in"=w764, "setup state"=w763, "Task number"=w762, "tdms file"=w761) -> ("error out"=w748:errorcluster, "setup state out"=w749:i32[], "Next task number"=w750:i32, "tdms file out"=w751:refnum<k34>)
                      n171 = call "merFISH_format_task_for_TDMS.vi"("Task"=w757, "error in"=w748, "setup state"=w749, "Task number"=w750, "tdms file"=w751) -> ("error out"=w747:errorcluster, "setup state out"=w746:i32[], "Next task number"=w745:i32, "tdms file out"=w744:refnum<k34>)
                      n172 = call "merFISH_format_task_for_TDMS.vi"("Task"=w784, "error in"=w747, "setup state"=w746, "Task number"=w745, "tdms file"=w744) -> ("error out"=w740:errorcluster, "setup state out"=w741:i32[], "Next task number"=w742:i32, "tdms file out"=w743:refnum<k34>)
                      n173 = call "merFISH_format_task_for_TDMS.vi"("Task"=w779, "error in"=w740, "setup state"=w741, "Task number"=w742, "tdms file"=w743) -> ("error out"=w753:errorcluster, "setup state out"=w754:i32[], "Next task number"=w755:i32, "tdms file out"=w756:refnum<k34>)
                    }
                    frame True {
                      n174 = To Variant(anything=w822) -> (Variant=w824:variant)
                      n175 = To Variant(anything=w819) -> (Variant=w821:variant)
                      n176 = To Variant(anything=w804) -> (Variant=w812:variant)
                      n177 = Bundle By Name(cluster=w817, "variant"=w824) -> (w823:T1)
                      n178 = Bundle By Name(cluster=w820, "variant"=w821) -> (w818:T1)
                      n179 = Bundle By Name(cluster=w798, "variant"=w812) -> (w806:T1)
                      n180 = call "merFISH_format_task_for_TDMS.vi"("Task"=w811, "error in"=w813, "setup state"=w814, "Task number"=w815, "tdms file"=w816) -> ("error out"=w810:errorcluster, "setup state out"=w809:i32[], "Next task number"=w808:i32, "tdms file out"=w807:refnum<k34>)
                      n181 = call "merFISH_format_task_for_TDMS.vi"("Task"=w806, "error in"=w810, "setup state"=w809, "Task number"=w808, "tdms file"=w807) -> ("error out"=w794:errorcluster, "setup state out"=w795:i32[], "Next task number"=w796:i32, "tdms file out"=w797:refnum<k34>)
                      n182 = call "merFISH_format_task_for_TDMS.vi"("Task"=w803, "error in"=w794, "setup state"=w795, "Task number"=w796, "tdms file"=w797) -> ("error out"=w790:errorcluster, "setup state out"=w791:i32[], "Next task number"=w792:i32, "tdms file out"=w793:refnum<k34>)
                      n183 = call "merFISH_format_task_for_TDMS.vi"("Task"=w823, "error in"=w790, "setup state"=w791, "Task number"=w792, "tdms file"=w793) -> ("error out"=w789:errorcluster, "setup state out"=w788:i32[], "Next task number"=w787:i32, "tdms file out"=w786:refnum<k34>)
                      n184 = call "merFISH_format_task_for_TDMS.vi"("Task"=w818, "error in"=w789, "setup state"=w788, "Task number"=w787, "tdms file"=w786) -> ("error out"=w799:errorcluster, "setup state out"=w800:i32[], "Next task number"=w801:i32, "tdms file out"=w802:refnum<k34>)
                    }
                  }
                }
                frame False {
                  n185 = To Variant(anything=w844) -> (Variant=w839:variant)
                  n186 = To Variant(anything=w842) -> (Variant=w837:variant)
                  n187 = Bundle By Name(cluster=w841, "variant"=w839) -> (w838:T1)
                  n188 = Bundle By Name(cluster=w843, "variant"=w837) -> (w836:T1)
                  n189 = call "merFISH_format_task_for_TDMS.vi"("Task"=w838, "error in"=w847, "setup state"=w845, "Task number"=w848, "tdms file"=w846) -> ("error out"=w828:errorcluster, "setup state out"=w829:i32[], "Next task number"=w830:i32, "tdms file out"=w831:refnum<k34>)
                  n190 = call "merFISH_format_task_for_TDMS.vi"("Task"=w836, "error in"=w828, "setup state"=w829, "Task number"=w830, "tdms file"=w831) -> ("error out"=w832:errorcluster, "setup state out"=w833:i32[], "Next task number"=w834:i32, "tdms file out"=w835:refnum<k34>)
                }
              }
            }
            n191 = To Variant(anything=TRUE) -> (Variant=w635:variant)
            n192 = To Variant(anything=FALSE) -> (Variant=w624:variant)
            n193 = To Variant(anything=0) -> (Variant=w682:variant)
            n194 = To Variant(anything=w605) -> (Variant=w606:variant)
            n195 = Bundle By Name(cluster=w621, "variant"=w635) -> (w622:T1)
            n196 = Bundle By Name(cluster=w621, "variant"=w624) -> (w616:T1)
            n197 = Bundle By Name(cluster=w681, "variant"=w682) -> (w676:T1)
            n198 = Bundle By Name(cluster=w599, "variant"=w606) -> (w604:T1)
            n199 = call "merFISH_format_task_for_TDMS.vi"("Task"=w604, "error in"=w600, "setup state"=w601, "Task number"=w602, "tdms file"=w603) -> ("error out"=w595:errorcluster, "setup state out"=w596:i32[], "Next task number"=w597:i32, "tdms file out"=w598:refnum<k34>)
            n200 = call "merFISH_format_task_for_TDMS.vi"("Task"=w611, "error in"=w595, "setup state"=w596, "Task number"=w597, "tdms file"=w598) -> ("error out"=w665:errorcluster, "setup state out"=w666:i32[], "Next task number"=w667:i32, "tdms file out"=w668:refnum<k34>)
            n201 = call "merFISH_format_task_for_TDMS.vi"("Task"=w676, "error in"=w665, "setup state"=w666, "Task number"=w667, "tdms file"=w668) -> ("error out"=w631:errorcluster, "setup state out"=w632:i32[], "Next task number"=w633:i32, "tdms file out"=w634:refnum<k34>)
            n202 = call "merFISH_format_task_for_TDMS.vi"("Task"=w622, "error in"=w631, "setup state"=w632, "Task number"=w633, "tdms file"=w634) -> ("error out"=w626:errorcluster, "setup state out"=w627:i32[], "Next task number"=w628:i32, "tdms file out"=w629:refnum<k34>)
            n203 = call "merFISH_format_task_for_TDMS.vi"("Task"=w625, "error in"=w626, "setup state"=w627, "Task number"=w628, "tdms file"=w629) -> ("error out"=w618:errorcluster, "setup state out"=w619:i32[], "Next task number"=w617:i32, "tdms file out"=w620:refnum<k34>)
            n204 = call "merFISH_format_task_for_TDMS.vi"("Task"=w616, "error in"=w618, "setup state"=w619, "Task number"=w617, "tdms file"=w620) -> ("error out"=w612:errorcluster, "setup state out"=w613:i32[], "Next task number"=w614:i32, "tdms file out"=w615:refnum<k34>)
            n205 = call "merFISH_format_task_for_TDMS.vi"("Task"=w611, "error in"=w612, "setup state"=w613, "Task number"=w614, "tdms file"=w615) -> ("error out"=w607:errorcluster, "setup state out"=w608:i32[], "Next task number"=w609:i32, "tdms file out"=w610:refnum<k34>)
            n206 = call "merFISH_format_task_for_TDMS.vi"("Task"=w669, "error in"=w607, "setup state"=w608, "Task number"=w609, "tdms file"=w610) -> ("error out"=w675:errorcluster, "setup state out"=w672:i32[], "Next task number"=w674:i32, "tdms file out"=w673:refnum<k34>)
          }
          n207 = call "merFISH_format_task_for_TDMS.vi"("Task"=w583, "error in"=w584, "setup state"=w576, "Task number"=w585, "tdms file"=w579) -> ("error out"=w582:errorcluster, "tdms file out"=w578:refnum<k34>)  [unwired: 2 out]
        }
      }
    }
    frame Error {
    }
  }
  n208 = TDMS List Contents(4:w21, 6:w19, 7:w20) -> (0:w27:errorcluster, 1:w24:string[], 3:w26:refnum<k34>)  [unwired: 1 out]
  n209 = Search 1D Array(1D array=w24, element=w18) -> (index of element=w25:i32)  [unwired: 1 in]
  n210 = Greater Or Equal To 0?(x=w25) -> (x >= 0?=w28:bool)
  n211 = case shown="False" w28 {
    tunnel: [w852 w860] -> w23
    tunnel: [w851 w859] -> w15
    tunnel: w26 -> [w852 w856]
    tunnel: w27 -> [w851 w855]
    tunnel: w18 -> [_ w854]
    tunnel: w19 -> [_ w853]
    frame False {
    }
    frame True {
      n212 = TDMS Close(8:w855, 11:w856) -> (0:w857:errorcluster, 3:w858:path)
      n213 = TDMS Delete Data(8:w857, 9:w854, 10:w853, 11:w858) -> (0:w862:errorcluster, 3:w863:path)  [unwired: 3 in]
      n214 = TDMS Open(8:w862, 10:T5."open" ("operation (0:open)"), 11:w863) -> (0:w859:errorcluster, 3:w860:refnum<k34>)  [unwired: 4 in]
    }
  }
  n215 = Build Array(u32 0) -> (w22:u32[])
  n216 = TDMS Write(0:w23, 5:w19, 7:w18, 9:w22, 11:w15) -> (4:w17:refnum<k34>, 15:→"error out":errorcluster)  [unwired: 1 in, 2 out]
  n217 = global write "Global_MAIN.vi" "tdms file out"(w17) -> ()
